vi "view class name.vi"(8 "error in":errorcluster, 11 "configuration in":refnum<class "NISE_CEF_serializable configuration.lvclass">) -> (0 "error out":errorcluster, 2 "view class":string, 3 "configuration out":refnum<class "NISE_CEF_serializable configuration.lvclass">)   [LabVIEW 2013, in "NISE_CEF_serializable configuration.lvclass"]
uses:
  NISE_CEF_serializable configuration.lvclass
  NISE_CEF_TreeControl.lvlib
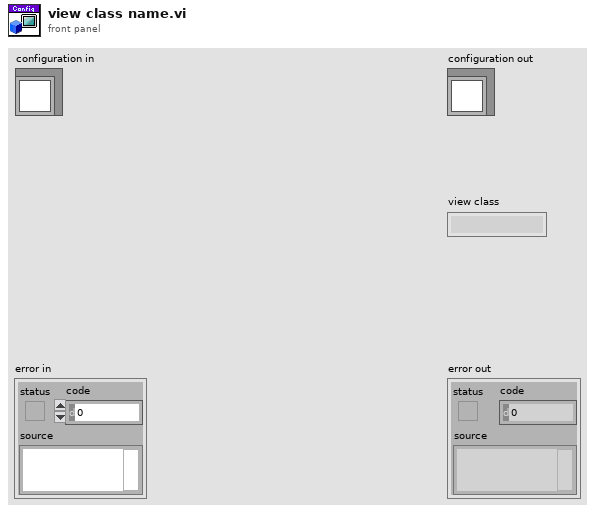
[diagram p1: front panel]
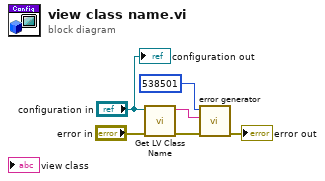
[diagram p0: block diagram]
diagram:
  n1 = call <vilib>:"Get LV Class Name.vi"("error in (no error)"="error in", "object"="configuration in") -> ("error out"=w4:errorcluster, "class name"=w3:string)  [unwired: 8 in]
  n2 = call "error generator.vi"("error in"=w4, "append error message"=w3, "error code (0)"=538501) -> ("error out"=→"error out":errorcluster)  [unwired: 6 in]
  "configuration out" <- "configuration in"
